vi "Dashboard Main.vi"() -> ()   [LabVIEW 2018]
uses:
  <vilib>/Rock Robotics/WPI/Camera/WPI_CameraExposure Values.ctl
  <vilib>/Rock Robotics/WPI/Camera/WPI_CameraWhite Balance Values.ctl
  <vilib>/Utility/miscctls.llb/LVRowAndColumnTypeDef.ctl
  <vilib>/event_ctls.llb/eventvkey.ctl
  <vilib>/Rock Robotics/Network Tables/NT Read Numeric Array.vi
  <vilib>/Rock Robotics/WPI/Dashboard/WPI_DashboardLogging Global.vi
panel:
  in  "Camera Settings Right":T1={"Frame Rate"=30, "Compression"=30, "Size"=1, "DB Camera Config"=FALSE} {"Frame Rate" scale=1.0..30.0; "Compression" scale=100.0..-1.0; "Size" items=["640x480", "320x240", "160x120"]}
  in  "Camera Name Right":string(combo)="No Camera Selection"
  out "Camera Perf":string
  in  "Camera Settings":T1={"Frame Rate"=30, "Compression"=30, "Size"=1, "DB Camera Config"=FALSE} {"Frame Rate" scale=1.0..30.0; "Compression" scale=100.0..-1.0; "Size" items=["640x480", "320x240", "160x120"]}
  in  "TCP":refnum<k5>
  in  "Rec Mode":enum32{"Stop", "Record", "Playback"}(radio)
  out "Robot IP":string
  out "Image Message":string="Timeout in Camera Communications"
  in  "Dashboard Tab":T2(tab)=enum."Camera"
  in  "Select Auto":string(combo)="Select Autonomous ..."
  out "NT Connection":bool
  out "MotorChart R":cluster{"Numeric":dbl, "Numeric":dbl}(graph)
  out "MotorChart L":cluster{"Numeric":dbl, "Numeric":dbl}(graph)
  out "MotorSliders R":cluster{"MotorSlide1":dbl, "MotorSlide2":dbl} {"MotorSlide2" scale=-1.0..1.0 scale format="%#_2e"; "MotorSlide1" scale=-1.0..1.0 scale format="%#_2e"}
  out "MotorSliders L":cluster{"MotorSlide1":dbl, "MotorSlide2":dbl} {"MotorSlide2" scale=-1.0..1.0 scale format="%#_2e"; "MotorSlide1" scale=-1.0..1.0 scale format="%#_2e"}
  out "Gyro":dbl(knob) scale=0.0..360.0
  out "JS1 Z":dbl(slide) scale=-1.0..1.0 scale format="%#_2e"
  out "JS1 Graph":cluster{"X":dbl, "Y":dbl}[](graph)
  out "JS1 Buttons":T3
  out "JS2 Z":dbl(slide) scale=-1.0..1.0 scale format="%#_2e"
  out "JS2 Graph":cluster{"X":dbl, "Y":dbl}[](graph)
  out "JS2 Buttons":T3
  out "Mode":T4(ring)=enum."Auto Disabled"
  out "Right Camera Perf":cluster{"Bandwidth (Mbps)":dbl, "FPS":dbl}
  out "Camera Image Right":T5(plugin-control)
  in  "DB/String 9":string
  in  "DB/String 8":string
  in  "DB/String 7":string
  in  "DB/String 6":string
  in  "DB/String 5":string
  in  "DB/String 4":string
  in  "DB/String 3":string
  in  "DB/String 2":string
  in  "DB/String 1":string
  in  "DB/String 0":string
  in  "DB/Slider 0":dbl(slide) scale=0.0..5.0
  in  "DB/Slider 1":dbl(slide) scale=0.0..5.0
  in  "DB/Slider 2":dbl(slide) scale=0.0..5.0
  in  "DB/Slider 3":dbl(slide) scale=0.0..5.0
  out "DB/LED 3":bool
  out "DB/LED 2":bool
  out "DB/LED 1":bool
  out "DB/LED 0":bool
  in  "DB/Button 3":bool
  in  "DB/Button 2":bool
  in  "DB/Button 1":bool
  in  "DB/Button 0":bool caption="New Name"
  in  "Camera Settings 3":T8={"Exposure"=enum."Auto", "Exposure (%)"=50.0, "Brightness"=20, "White Balance"=enum."Auto", "Color Temp (K)"=0.0} {"Brightness" min=0 max=100}
  in  "Camera Settings 2":T8={"Exposure"=enum."Auto", "Exposure (%)"=50.0, "Brightness"=20, "White Balance"=enum."Auto", "Color Temp (K)"=0.0} {"Brightness" min=0 max=100}
  in  "Hatch Mover Scale":dbl=0.4 min=0.0 max=1.0 step=0.1
  in  "Elevator Scale":dbl=0.5 min=0.0 max=1.0 step=0.1
  in  "Autonomous Wait":u32=10
  in  "Hatch Extend Setpoint":dbl=0.4 min=0.0 max=1.0 step=0.1 format="%#_1g"
  in  "Hatch Extend Duration":dbl=10.0 min=0.0 max=50.0 step=0.1
  in  "Ball Stop I":dbl=10.0 min=0.0 max=50.0 step=0.1
  in  "Ball Hold Time":dbl=1.0 min=0.0 max=1000.0 step=1.0
  in  "Pivot Left":dbl=0.20000000000000004 min=0.0 max=1.0 step=0.1 format="%#_1g"
  in  "Pivot Right":dbl=0.20000000000000004 min=0.0 max=1.0 step=0.1
  in  "Elevator":dbl=0.7000000000000001 min=0.0 max=1.0 step=0.1 format="%#_3g"
  in  "Elevator Time":dbl=2.0 min=0.0 step=0.1
  in  "Ball":dbl=1.0 min=0.0 max=1.0 step=0.1
  in  "Cheezy Dr Mode":u32=2 max=2 step=1
  in  "MaxSpeedSlow":dbl=0.7
  in  "SlowRate":dbl=1.0
  in  "MaxTurnSlow":dbl=0.65
  in  "MaxTurnRateSlow":dbl=10.0
  in  "SlowModeSettings":i32=2
  in  "Elevator Ball 1":dbl=2.0
  in  "Elevator Ball 2":dbl=2.0
  in  "Elevator Ball 3":dbl=2.0
  in  "Elevator Hatch 1":dbl=2.0
  in  "Elevator Hatch 2":dbl=2.0
  in  "Elevator Hatch 3":dbl=2.0
  in  "Elevator Cargo":dbl=2.0
  in  "Test Slider":dbl(slide) scale=0.0..100.0 scale format="%#_3g"
  in  "On/Off":bool caption="Solenoid"
  in  "Test Name":u16(ring) items=["Select the test to run..."]
  in  "Test Tree":string(tree)
  in  "Motor":cluster{"Value":dbl, "Enable":bool} {"Value" scale=-1.0..1.0 scale format="%#_3g"}
  out "Progress":T9 {"Test Progress" scale=0.0..100.0}
  in  "Rev/Fwd":cluster{"Forward":bool, "Reverse":bool}
  in  "Test Ring":u16(ring) items=["Monochrome", "Color"]
  out "Cmd Status":string
  in  "Execute Command":bool
  in  "Command Params":string[][](table)
  in  "Command Selection":i32(listbox)
  in  "CheckList":i32(listbox)
  out "Tree":string(tree)
  out "Results":T10(array[cluster]) {"Score" format="%#_3g"; "Pixels"."Rectangle"."Numeric 5" format="%#_3g"; "Pixels"."Rectangle"."Numeric 3" format="%#_3g"; "Pixels"."Rectangle"."Numeric 2" format="%#_3g"; "Pixels"."Rectangle"."Numeric" format="%#_3g"; "Normalized"."Rectangle"."Numeric 5" format="%#_2g"; "Normalized"."Rectangle"."Numeric 3" format="%#_2g"; "Normalized"."Rectangle"."Numeric 2" format="%#_2g"; "Normalized"."Rectangle"."Numeric" format="%#_2g"; "Normalized"."Center"."?" format="%#_3g"; "Normalized"."Center"."?" format="%#_3g"; "Distance (ft)" format="%#_3g"}
  out "Camera Image":T5(plugin-control)
  out "Background":bool
  in  "Camera Name":string(combo)="No Camera Selection"
  # "HW"
  # "HW"
  # "Joysticks"
  # "Drive Motors"
  # "Front"
  # "Right"
  # "Left"
  # "Back"
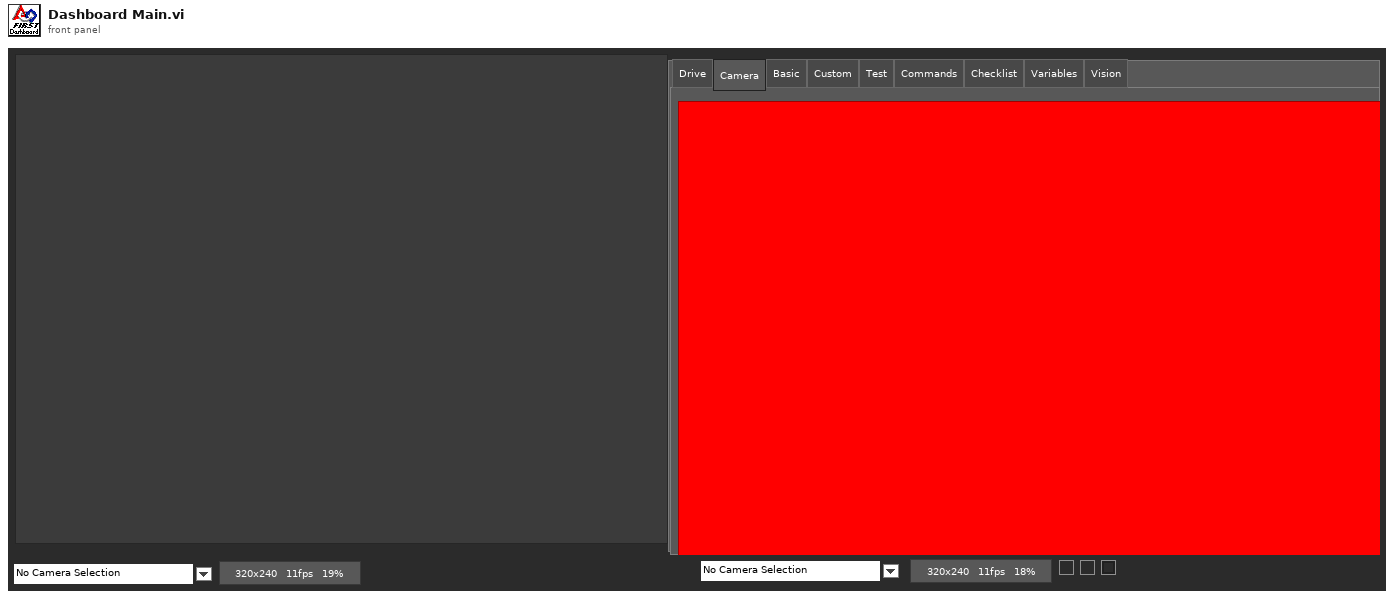
[diagram p1: front panel]
types:
  T1 = cluster{"Frame Rate":i32, "Compression":i32, "Size":u16, "DB Camera Config":bool}
  T2 = enum32{"Drive", "Camera", "Basic", "Custom", "Test", "Commands", "Checklist", "Variables", "Vision"}
  T3 = cluster{bool, bool, bool, bool, bool, bool, bool, bool, bool, bool, bool, bool}
  T4 = enum8{"Tele-Op Disabled", "Tele-Op Enabled", "Auto Disabled", "Auto Enabled", "Test Disabled", "Test Enabled", "Disconnected", "No Code", "E-Stop"}
  T5 = typedef "IMAQ Image.ctl" = refnum<image>
  T6 = typedef "WPI_CameraExposure Values.ctl" = enum16{"Auto", "Flicker-free 50 Hz", "Flicker-free 60 Hz", "Hold current", "Custom"}
  T7 = typedef "WPI_CameraWhite Balance Values.ctl" = enum16{"Auto", "Fixed indoor", "Fixed outdoor 1", "Fixed outdoor 2", "Fixed fluorescent 1", "Fixed fluorescent 2", "Hold current", "Custom"}
  T8 = cluster{"Exposure":T6, "Exposure (%)":dbl, "Brightness":i32, "White Balance":T7, "Color Temp (K)":dbl}
  T9 = cluster{"Test Progress":u8, "Test Progress Text":string}
  T10 = cluster{"Distance (ft)":dbl, "Score":dbl, "Normalized":cluster{"Center":cluster{dbl, dbl}, "Rectangle":cluster{"Numeric":dbl, "Numeric 2":dbl, "Numeric 3":dbl, "Numeric 5":dbl}}, "Pixels":cluster{"Center":cluster{dbl, dbl}, "Rectangle":cluster{"Numeric":dbl, "Numeric 2":dbl, "Numeric 3":dbl, "Numeric 5":dbl}}}[]
  T11 = typedef "Image Type" = u32
  T12 = cluster{"Save Path":path, "Interval (s)":dbl, "Keep":i32}
  T13 = enum32{"Drive", "Camera", "Basic", "Custom", "Test", "Commands", "Checklist", "Variables"}
  T14 = cluster{"IDs":cluster{"RPC field ID":u16, "Unique ID":u16}, "String":string}
  T15 = cluster{"Error Strings":string, "Disable Counts":cluster{u16, u16}, "Rail Faults":cluster{u16, u16, u16}, "Robot IP":string, "DB Mode":u8, "Event Info":cluster{"Name":string, "Type":u8, "Number":u16, "Replay":u8}}
  T16 = cluster{"Storage":cluster{"Disk Free":u64, "RAM Block":u32, "RAM free":u32}, "CPU Utilization":cluster{"CPU % ISR":sgl, "CPU % Time Crit":sgl, "CPU % Timed Str":sgl, "CPU % High":sgl, "CPU % Above":sgl, "CPU % Normal":sgl, "CPU % Low":sgl}, "CAN":cluster{"% Bus Utilization":sgl, "Bus Off Cnt":u32, "TX_FIFO Full Cnt":u32, "Receive Error Cnt":u8, "Transmit Error Cnt":u8}, "HID":cluster{"HID Outputs":u32, "Rumble Low":u16, "Rumble High":u16}[]}
  T17 = cluster{"Status bits":cluster{"Test Mode":bool, "Autonomous":bool, "Enabled":bool, "Code Start":bool, "Brownout":bool, "Reserved 2":bool, "Reserved 3":bool, "E-Stop":bool}, "Code Trace":cluster{"Disabled":bool, "TeleOp":bool, "Auto":bool, "Test":bool}, "Controller Type":enum16{"unknown", "cRIO", "roboRio"}, "Code?":enum16{"unknown", "noCode", "code"}, "Battery V":dbl}
  T18 = cluster{"Control Bits":cluster{"TestMode":bool, "Autonomous":bool, "Enabled":bool, "FMS Present":bool, bool, bool, bool, "E-Stop":bool}, "Team Station ":u8, "Countdown":sgl, "Joystick Values":cluster{"Axes":dbl[], "Buttons":bool[], "POVs":i16[]}[]}
  T19 = cluster{"Axes":dbl[], "Buttons":bool[], "POVs":i16[]}[]
  T20 = cluster{"Axes":dbl[], "Buttons":bool[], "POVs":i16[]}
  T21 = cluster{"Buttons[0]":bool, "Buttons[1]":bool, "Buttons[2]":bool, "Buttons[3]":bool, "Buttons[4]":bool, "Buttons[5]":bool, "Buttons[6]":bool, "Buttons[7]":bool, "Buttons[8]":bool, "Buttons[9]":bool, "Buttons[10]":bool, "Buttons[11]":bool}
  T22 = cluster{"Camera Image":refnum<vi>, "Dashboard Tab":refnum<vi>, "Background":refnum<vi>, "Rec Mode":refnum<vi>, "Test Slider":refnum<vi>, "On/Off ":refnum<vi>, "Test Ring":refnum<vi>, "Rev/Fwd":refnum<vi>, "Test Name":refnum<vi>, "Motor":refnum<vi>, "Progress":refnum<vi>, "CheckList":refnum<vi>, "Tree":refnum<vi>, "Test Tree":refnum<vi>, "Command Params":refnum<vi>, "Command Selection":refnum<vi>, "Execute Command":refnum<vi>, "Cmd Status":refnum<vi>, "Camera Settings":refnum<vi>, "Camera Name":refnum<vi>, "Camera Perf":refnum<vi>, "Camera Settings Right":refnum<vi>, "Camera Name Right":refnum<vi>, "Camera Image Right":refnum<vi>}
  T23 = cluster{"Global Rectangle":i32[], "Contours":cluster{"Contour Type":u32, "ROI Type":u32, "Points":i32[]}[]}
  T24 = cluster{"Camera Name":string, string, "Saved DB Images Info":cluster{"Save Path":path, "Interval (s)":dbl, "Keep":i32}}
  T25 = cluster{"Camera Name Right":string, string, "Saved DB Images Info":cluster{"Save Path":path, "Interval (s)":dbl, "Keep":i32}}
  T26 = cluster{"Operation":enum16{"Update", "Clear"}, "Color Box":u32}[]
  T27 = typedef "eventvkey.ctl" = enum16{"ASCII", "Enter", "Return", "Shift", "Ctrl", "Alt", "Cmd", "Opt", "Caps", "NumLock", "Clear", "Break", "Up", "Down", "Left", "Right", "Insert", "Delete", "Home", "End", "PageUp", "PageDown", "Escape", "Help", "Pause", "ScrollLock", "F1", "F2", "F3", "F4", "F5", "F6", "F7", "F8", "F9", "F10", "F11", "F12", "F13", "F14", "F15", "F16", "F17", "F18", "F19", "F20", "F21", "F22", "F23", "F24", "Play", "VolumeUp", "VolumeDown", "Mute", "Two Byte Char"}
  T28 = cluster{"Image Size":bool, "Image Type":bool, "Pixel Value":bool, "ROI Information":bool, "Zoom Factor":bool}
  T29 = cluster{"Operation":enum16{"Update", "Clear"}, "Color Box":u32}
  T30 = typedef "LVRowAndColumnTypeDef.ctl" = cluster{"Row":i32, "Column":i32}
  T31 = cluster{"Shift":bool, "Ctrl":bool, "Alt":bool, "Cmd":bool, "Opt":bool}
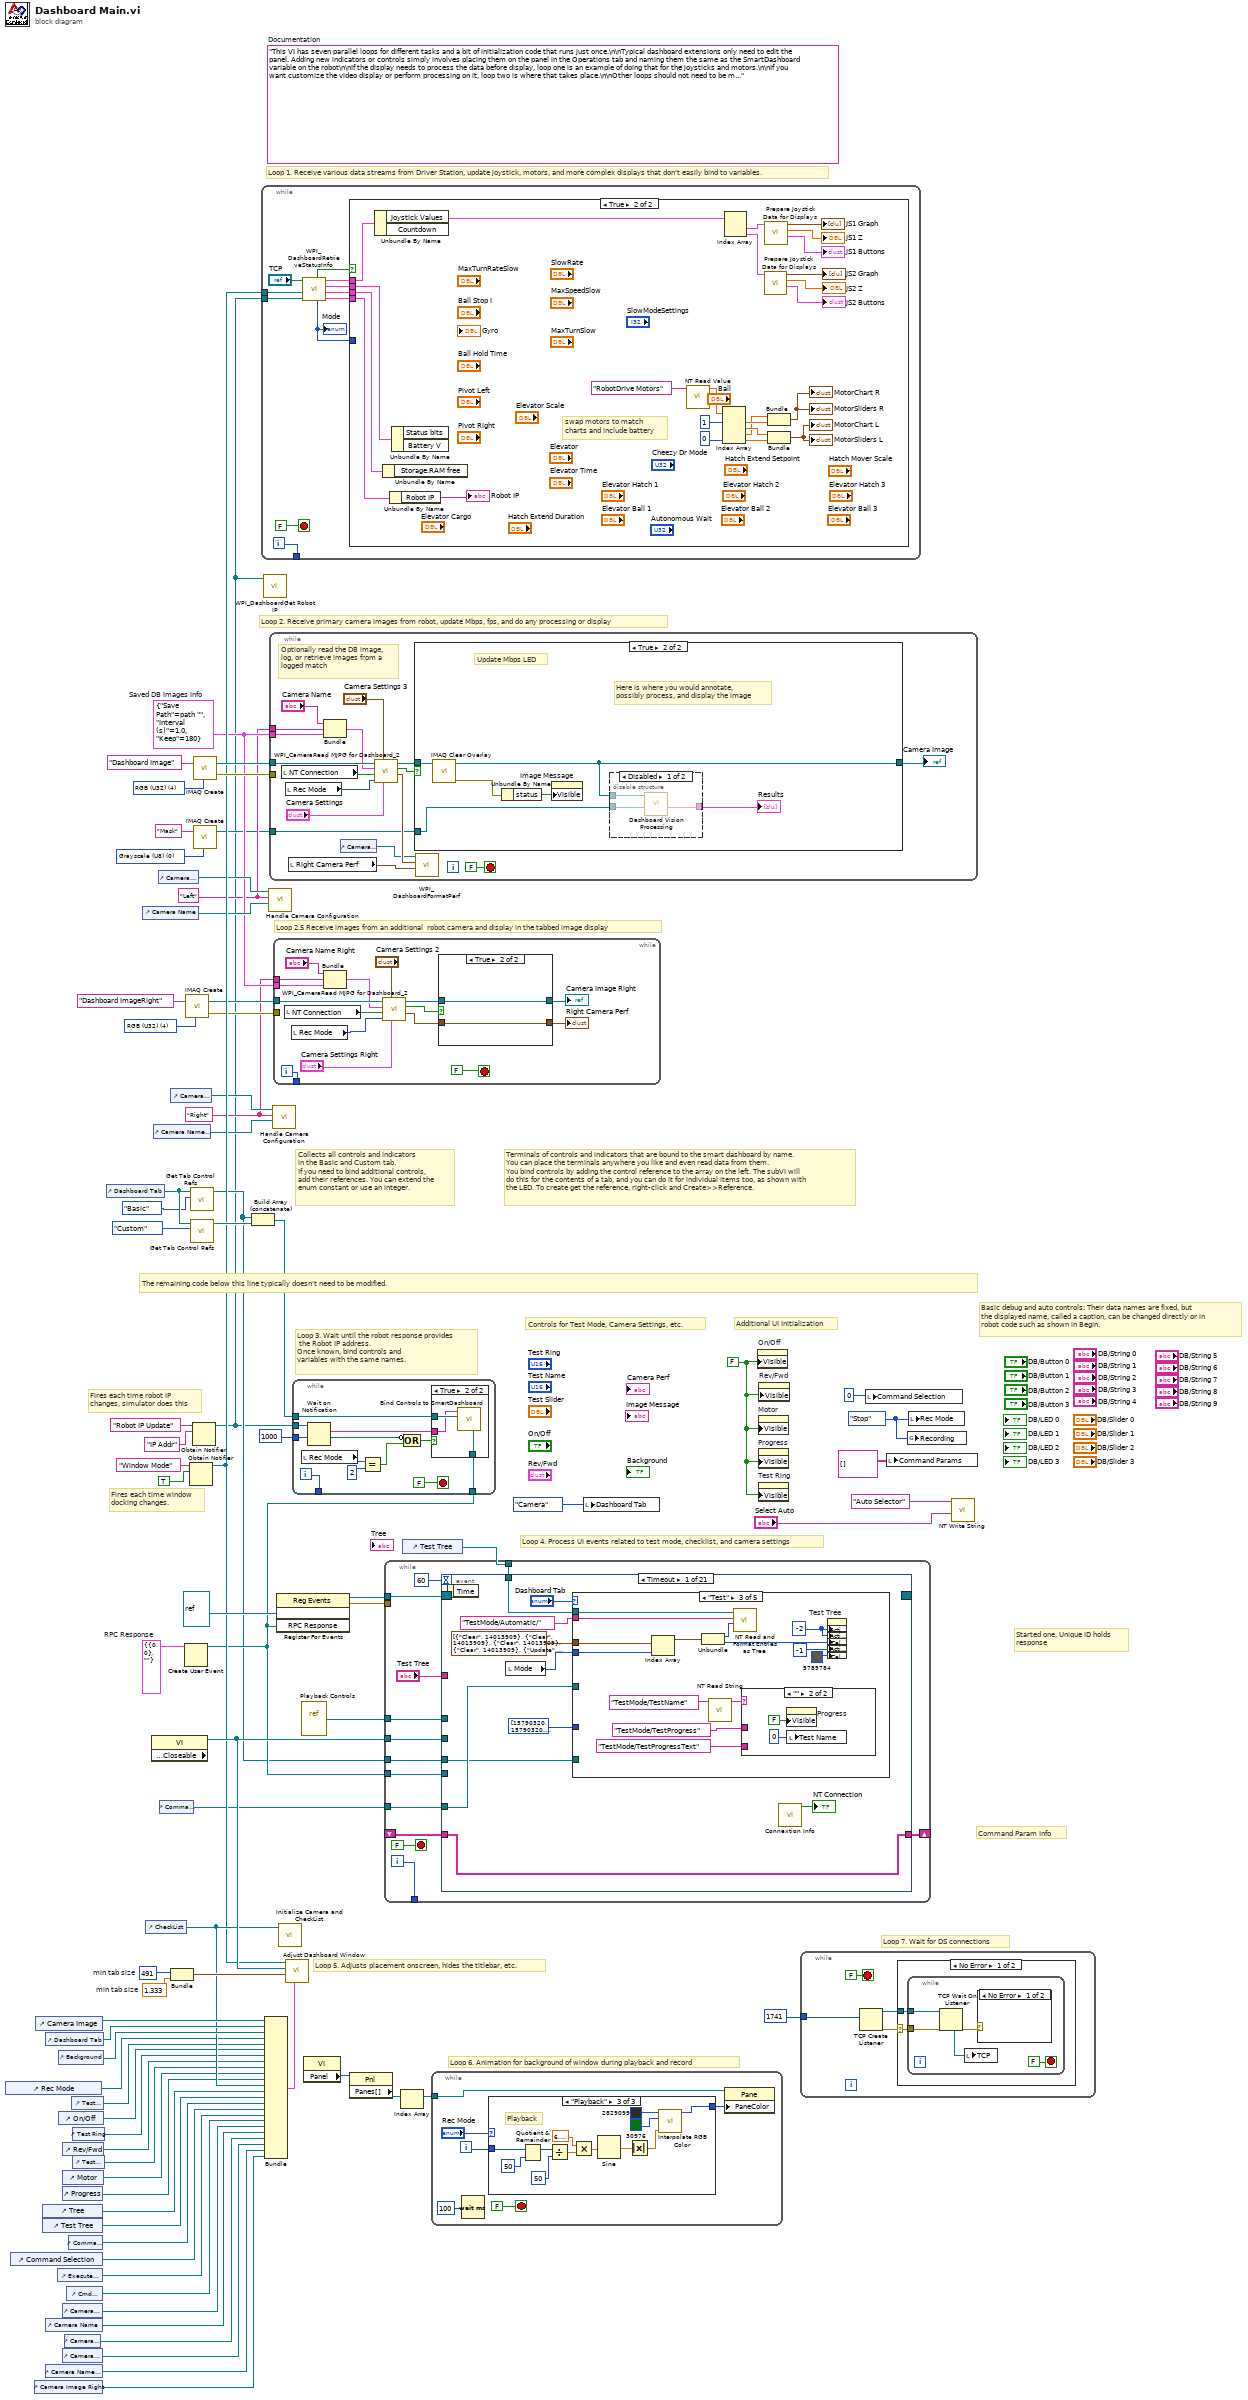
[diagram p0: block diagram]
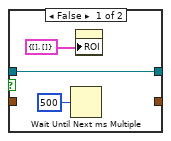
[diagram p2: hidden frame]
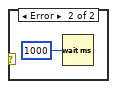
[diagram p3: hidden frame]
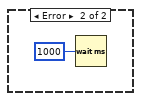
[diagram p4: hidden frame]
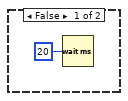
[diagram p5: hidden frame]
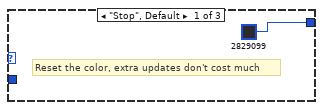
[diagram p6: hidden frame]
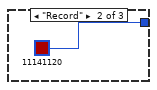
[diagram p7: hidden frame]
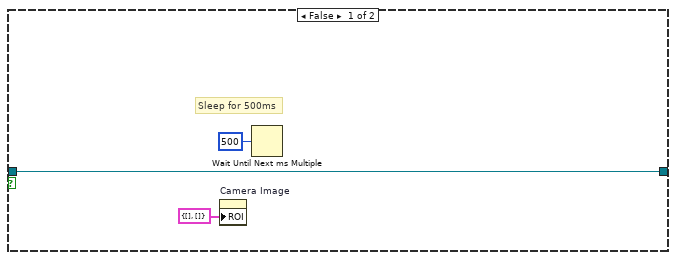
[diagram p9: hidden frame]
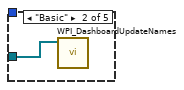
[diagram p12: hidden frame]
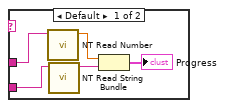
[diagram p13: hidden frame]
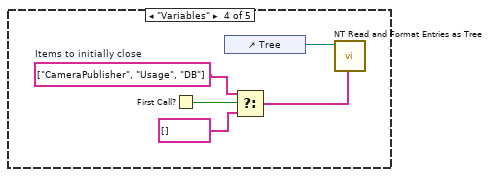
[diagram p14: hidden frame]
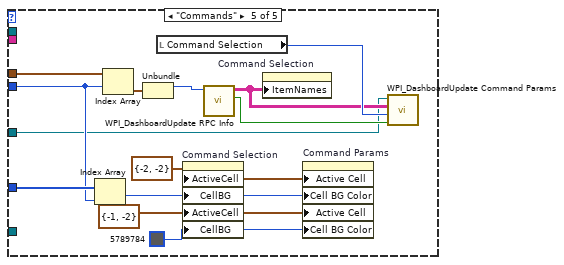
[diagram p15: hidden frame]
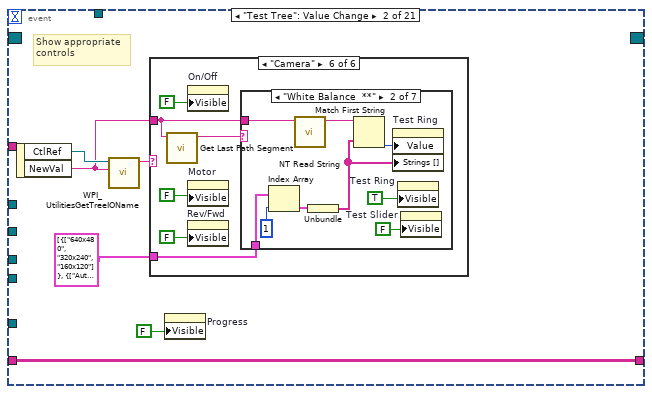
[diagram p16: hidden frame]
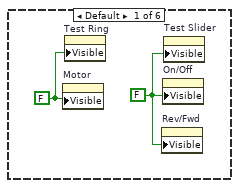
[diagram p17: hidden frame]
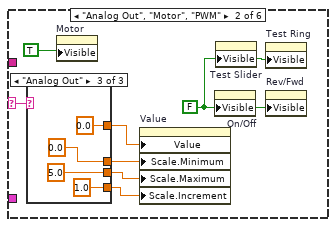
[diagram p18: hidden frame]
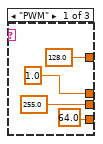
[diagram p19: hidden frame]
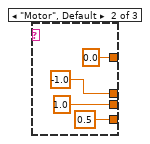
[diagram p20: hidden frame]
diagram:
  w3 = T11 0 items=["Grayscale (U8)", "Grayscale (I16)", "Grayscale (SGL)", "Complex (CSG)", "RGB (U32)", "HSL (U32)", "RGB (U64)"] ("Image Type")
  w7 = T12 {"Save Path"=path "", "Interval (s)"=1.0, "Keep"=180}  # Saved DB Images Info
  w6 = "Right"
  w5 = "Left"
  w17 = T11 4 items=["Grayscale (U8)", "Grayscale (I16)", "Grayscale (SGL)", "Complex (CSG)", "RGB (U32)", "HSL (U32)", "RGB (U64)"] ("Image Type")
  w33 = T14 {"IDs"={"RPC field ID"=0, "Unique ID"=0}, "String"=""}  # RPC Response
  w55 = 491  # min tab size
  w54 = 1.333  # min tab size
  w62 = enum32{"Stop", "Record", "Playback"}."Stop" ("Rec Mode")
  w39 = FALSE ("Visible")
  (unwired) "This VI has seven parallel loops for different tasks and a bit of initialization code that runs just once.\n\nTypical dashboard extensions only need to edit the panel. Adding new indicators or controls simply involves placing them on the panel in the Operations tab and naming them the same as the SmartDashboard variable on the robot\n\nIf the display needs to process the data before display, loop one is an example of doing that for the joysticks and motors.\n\nIf you want customize the video display or perform processing on it, loop two is where that takes place.\n\nOther loops should not need to be modified. They are pretty standard, and document the task they perform."  # Documentation
  w79 = T11 4 items=["Grayscale (U8)", "Grayscale (I16)", "Grayscale (SGL)", "Complex (CSG)", "RGB (U32)", "HSL (U32)", "RGB (U64)"] ("Image Type")
  # "Loop 2.5 Receive images from an additional  robot camera and display in the tabbed image display"
  # "Command Param Info"
  # "Started one, Unique ID holds\nresponse"
  # "Loop 7. Wait for DS connections"
  # "Basic debug and auto controls: Their data names are fixed, but\nthe displayed name, called a caption, can be changed directly or in\nrobot code such as shown in Begin."
  # "Controls for Test Mode, Camera Settings, etc."
  # "Additional UI Initialization"
  # "Loop 6. Animation for background of window during playback and record"
  # "Fires each time robot IP\nchanges, simulator does this"
  # "Fires each time window\ndocking changes."
  # "Collects all controls and indicators\nin the Basic and Custom tab.\nIf you need to bind additional controls,\nadd their references. You can extend the\nenum constant or use an integer."
  # "The remaining code below this line typically doesn't need to be modified."
  # "Loop 4. Process UI events related to test mode, checklist, and camera settings"
  # "Terminals of controls and indicators that are bound to the smart dashboard by name.\nYou can place the terminals anywhere you like and even read data from them.\nYou bind controls by adding the control reference to the array on the left. The subVI will\ndo this for the contents of a tab, and you can do it for individual items too, as shown with\nthe LED. To create get the reference, right-click and Create>>Reference."
  # "Loop 3. Wait until the robot response provides\n the Robot IP address.\nOnce known, bind controls and\nvariables with the same names."
  # "Loop 5. Adjusts placement onscreen, hides the titlebar, etc."
  # "Loop 1. Receive various data streams from Driver Station, update joystick, motors, and more complex displays that don't easily bind to variables."
  # "Loop 2. Receive primary camera images from robot, update Mbps, fps, and do any processing or display"
  n1 = control-ref of="Rec Mode"() -> (w45:refnum<vi>)
  n2 = control-ref of="Command Selection"() -> (w32:refnum<vi>)
  n3 = control-ref of="Camera Image Right"() -> (w10:refnum<vi>)
  n4 = control-ref of="Camera Image"() -> (w57:refnum<vi>)
  n5 = control-ref of="Tree"() -> (w49:refnum<vi>)
  n6 = control-ref of="Test Tree"() -> (w48:refnum<vi>)
  n7 = control-ref of="Dashboard Tab"() -> (w56:refnum<vi>)
  n8 = control-ref of="Camera Name"() -> (w23:refnum<vi>)
  n9 = control-ref of="Camera Name Right"() -> (w11:refnum<vi>)
  n10 = control-ref of="Execute Command"() -> (w34:refnum<vi>)
  n11 = control-ref of="Background"() -> (w52:refnum<vi>)
  n12 = control-ref of="On/Off"() -> (w43:refnum<vi>)
  n13 = control-ref of="Progress"() -> (w40:refnum<vi>)
  n14 = control-ref of="Camera Settings"() -> (w24:refnum<vi>)
  n15 = control-ref of="Camera Settings Right"() -> (w12:refnum<vi>)
  n16 = control-ref of="Rev/Fwd"() -> (w41:refnum<vi>)
  n17 = control-ref of="Motor"() -> (w46:refnum<vi>)
  n18 = control-ref of="Camera Perf"() -> (w22:refnum<vi>)
  n19 = control-ref of="Cmd Status"() -> (w28:refnum<vi>)
  n20 = control-ref of="Command Params"() -> (w35:refnum<vi>)
  n21 = control-ref of="Test Slider"() -> (w44:refnum<vi>)
  n22 = control-ref of="Test Ring"() -> (w42:refnum<vi>)
  n23 = control-ref of="Test Name"() -> (w47:refnum<vi>)
  n24 = control-ref of="Dashboard Tab"() -> (w60:refnum<vi>)
  n25 = control-ref of="Camera Name"() -> (w25:refnum<vi>)
  n26 = control-ref of="CheckList"() -> (w50:refnum<vi>)
  n27 = property class="VI" props=["Front Panel.Closeable"]() -> (reference out=w61:refnum<vi>)  [unwired: 2 in, 2 out]
  n28 = control-ref of="Camera Name Right"() -> (w13:refnum<vi>)
  n29 = control-ref of="Camera Settings"() -> (w26:refnum<vi>)
  n30 = control-ref of="Command Params"() -> (w27:refnum<vi>)
  n31 = control-ref of="Camera Settings Right"() -> (w14:refnum<vi>)
  n32 = Bundle("min tab size"=w55, "min tab size"=w54) -> (w53:cluster{"min tab size":i32, "min tab size":dbl})  [unwired: 1 in]
  n33 = Create User Event(user event datatype=w33) -> (user event=w29:refnum<user-event>)  [unwired: 1 in, 1 out]
  n34 = call "IMAQ Create"("Image Name"="Dashboard ImageRight", "Image Type"=w17) -> ("New Image"=w16:T5, "error out"=w15:errorcluster)  [unwired: 2 in, 1 out]
  n35 = Obtain Notifier(name (unnamed)="Window Mode", notification data type=TRUE) -> (notifier out=w38:refnum<notifier>)  [unwired: 2 in, 2 out]
  n36 = call <vilib>:"Get Tab Control Refs.vi"("Page Index"=T13."Basic" ("Dashboard Tab"), "TabControl in"=w60) -> ("ControlsOnPage"=w21:refnum<vi>[])  [unwired: 9 in]
  n37 = call <vilib>:"Get Tab Control Refs.vi"("Page Index"=T13."Custom" ("Dashboard Tab"), "TabControl in"=w60) -> ("ControlsOnPage"=w59:refnum<vi>[])  [unwired: 9 in]
  n38 = Obtain Notifier(name (unnamed)="Robot IP Update", notification data type="IP Addr" ("name (unnamed)")) -> (notifier out=w1:refnum<notifier>)  [unwired: 2 in, 2 out]
  n39 = call "IMAQ Create"("Image Name"="Dashboard Image", "Image Type"=w79) -> ("New Image"=w77:T5, "error out"=w76:errorcluster)  [unwired: 2 in, 1 out]
  n40 = call "IMAQ Create"("Image Name"="Mask", "Image Type"=w3) -> ("New Image"=w2:T5)  [unwired: 2 in, 2 out]
  n41 = Build Array (concatenate)(w21, w59) -> (w58:refnum<vi>[])
  n42 = while {
    tunnel: [w89] -> _
    tunnel: w1 -> [w83]
    tunnel: w38 -> [w80]
    i -> [w89]
    stop <- FALSE stop-if-true
    n43 = call <vilib>:"WPI_DashboardRetrieveStatusInfo.vi"("Binding Refnum"=w83, "Window Mode Notifier"=w80, "TCP Cnx"="TCP") -> ("Power and Errors"=w84:T15, "Robot Metrics"=w87:T16, "Status Info"=w88:T17, "Control Info"=w85:T18, "Robot Mode"=w82:T4, "Process?"=w86:bool)  [unwired: 3 in]
    "Mode" <- w82
    n44 = case shown="True" w86 {
      tunnel: w88 -> [_ w115]
      tunnel: w87 -> [_ w114]
      tunnel: w85 -> [_ w113]
      tunnel: w84 -> [_ w112]
      tunnel: w82 -> [_ _]
      frame False {
        n45 = Wait (ms)(milliseconds to wait=u32 20) -> ()  [unwired: 1 out]
      }
      frame True {
        # "swap motors to match\ncharts and include battery"
        n46 = Unbundle By Name(w113) -> ("Joystick Values"=w103:T19)  [unwired: 1 out]
        n47 = Unbundle By Name(w114) -> ()  [unwired: 1 out]
        n48 = Unbundle By Name(w112) -> ("Robot IP"=→"Robot IP":string)
        n49 = Unbundle By Name(w115) -> ()  [unwired: 2 out]
        n50 = call-poly <vilib>:"NT Read Value.vi"("Name"="RobotDrive Motors") -> ("Numeric Array"=w93:dbl[])  [unwired: 9 in, 1 out]
        n51 = Index Array(array=w93, index #1=1, index #4=0) -> (element #1=w107:dbl, element #2=w108:dbl, element #3=w106:dbl, element #4=w111:dbl)  [unwired: 2 in]
        n52 = Index Array(array=w103) -> (element #1=w102:T20, element #2=w98:T20)  [unwired: 2 in]
        n53 = call "Prepare Joystick Data for Displays.vi"("Joystick Values"=w98) -> ("Buttons"=→"JS2 Buttons":T21, "Z Axis"=→"JS2 Z":dbl, "Cartesian Data"=→"JS2 Graph":cluster{"X axis":dbl, "X axis":dbl}[])  [unwired: 8 in]
        n54 = call "Prepare Joystick Data for Displays.vi"("Joystick Values"=w102) -> ("Buttons"=→"JS1 Buttons":T21, "Z Axis"=→"JS1 Z":dbl, "Cartesian Data"=→"JS1 Graph":cluster{"X axis":dbl, "X axis":dbl}[])  [unwired: 8 in]
        n55 = Bundle("Numeric"=w106, "Numeric"=w107) -> (→"MotorChart R" →"MotorSliders R":cluster{"Numeric":dbl, "Numeric":dbl})  [unwired: 1 in]
        n56 = Bundle("Numeric"=w108, "Numeric"=w111) -> (→"MotorChart L" →"MotorSliders L":cluster{"Numeric":dbl, "Numeric":dbl})  [unwired: 1 in]
      }
    }
  }
  n57 = call <vilib>:"WPI_DashboardGet Robot IP.vi"("Notifier in"=w1) -> ()  [unwired: 11 in]
  n58 = Bundle("Camera Image"=w57, "Dashboard Tab"=w56, "Background"=w52, "Rec Mode"=w45, "Test Slider"=w44, "On/Off"=w43, "Test Ring"=w42, "Rev/Fwd"=w41, "Test Name"=w47, "Motor"=w46, "Progress"=w40, "CheckList"=w50, "Tree"=w49, "Test Tree"=w48, "Command Params"=w35, "Command Selection"=w32, "Execute Command"=w34, "Cmd Status"=w28, "Camera Settings"=w24, "Camera Name"=w23, "Camera Perf"=w22, "Camera Settings Right"=w12, "Camera Name Right"=w11, "Camera Image Right"=w10) -> (w51:T22)  [unwired: 1 in]
  n59 = call "Handle Camera Configuration.vi"("CameraNameRef"=w25, "Display Name"=w5, "ClusterRef"=w26) -> ()  [unwired: 9 in]
  n60 = while {
    tunnel: w77 -> [w131]
    tunnel: w76 -> [_]
    tunnel: w7 -> [w124]
    tunnel: w5 -> [w121]
    tunnel: w2 -> [w117]
    stop <- FALSE stop-if-true
    # "Optionally read the DB image,\nlog, or retrieve images from a\nlogged match"
    n61 = local read "NT Connection"() -> (w125:bool)
    n62 = local read "Rec Mode"() -> (w128:enum32{"Stop", "Record", "Playback"})
    n63 = local read "Right Camera Perf"() -> (w119:cluster{"Bandwidth (Mbps)":dbl, "FPS":dbl})
    n64 = Bundle("Camera Name"="Camera Name", w121, "Saved DB Images Info"=w124) -> (w123:T24)  [unwired: 1 in]
    n65 = control-ref of="Camera Perf"() -> (w118:refnum<vi>)
    n66 = call <vilib>:"WPI_CameraRead MJPG for Dashboard_2.vi"("Camera Settings"="Camera Settings", "Camera Settings 2"="Camera Settings 3", "Rec Mode"=w128, "NT Connection"=w125, "Capture Info"=w123, "Image in"=w131) -> ("perf info"=w120:cluster{"Bandwidth (Mbps)":dbl, "fps":dbl}, "Active"=w129:bool, "Image\\ out"=w130:T5)  [unwired: 3 in]
    n67 = case shown="True" w129 {
      tunnel: w130 -> [w134 w139]
      tunnel: [w134 w138] -> w126
      tunnel: w117 -> [_ w137]
      frame False {
        # "Sleep for 500ms"
        n68 = property on="Camera Image" class="ImageControl"("ROI"=T23 {"Global Rectangle"=[], "Contours"=[]}) -> ()  [unwired: 2 in, 2 out]
        n69 = Wait Until Next ms Multiple(millisecond multiple=u32 500) -> ()  [unwired: 1 out]
      }
      frame True {
        # "Here is where you would annotate,\npossibly process, and display the image"
        # "Update Mbps LED"
        n70 = call "IMAQ Clear Overlay"("Image"=w139) -> ("error out"=w140:errorcluster, "Image Out"=w138:T5)  [unwired: 2 in, 7 out]
        n71 = Unbundle By Name(w140) -> ("status"=w141:bool)
        n72 = property on="Image Message" class="Str"("Visible"=w141) -> ()  [unwired: 2 in, 2 out]
        n73 = disable-structure shown="Disabled" {
          disable-tunnel: w138 -> [w144 _]
          disable-tunnel: w137 -> [w143 _]
          disable-tunnel: [w142 _] -> w136
          frame Disabled {
            n74 = call "Dashboard Vision Processing.vi"("Image 2"=w143, "Image"=w144) -> ("Results"=w142:T10)  [unwired: 8 in, 1 out]
          }
          frame Enabled {
          }
        }
        "Results" <- w136
      }
    }
    "Camera Image" <- w126
    n75 = call <vilib>:"WPI_DashboardFormatPerf.vi"("Right Camera Perf"=w119, "Performance"=w120, "String in"=w118) -> ()  [unwired: 9 in]
  }
  n76 = call "Handle Camera Configuration.vi"("CameraNameRef"=w13, "Display Name"=w6, "ClusterRef"=w14) -> ()  [unwired: 9 in]
  n77 = while {
    tunnel: w16 -> [w160]
    tunnel: w15 -> [_]
    tunnel: [w155] -> _
    tunnel: w7 -> [w151]
    tunnel: w6 -> [w148]
    i -> [w155]
    stop <- FALSE stop-if-true
    n78 = local read "NT Connection"() -> (w152:bool)
    n79 = local read "Rec Mode"() -> (w159:enum32{"Stop", "Record", "Playback"})
    n80 = Bundle("Camera Name Right"="Camera Name Right", w148, "Saved DB Images Info"=w151) -> (w150:T25)  [unwired: 1 in]
    n81 = call <vilib>:"WPI_CameraRead MJPG for Dashboard_2.vi"("Camera Settings"="Camera Settings Right", "Camera Settings 2"="Camera Settings 2", "Rec Mode"=w159, "NT Connection"=w152, "Capture Info"=w150, "Image in"=w160) -> ("perf info"=w146:cluster{"Bandwidth (Mbps)":dbl, "fps":dbl}, "Active"=w154:bool, "Image\\ out"=w157:T5)  [unwired: 3 in]
    n82 = case shown="True" w154 {
      tunnel: w157 -> [w162 w165]
      tunnel: [w162 w165] -> w153
      tunnel: [_ w164] -> w147
      tunnel: w146 -> [_ w164]
      frame False {
        n83 = Wait Until Next ms Multiple(millisecond multiple=u32 500) -> ()  [unwired: 1 out]
        n84 = property on="Camera Image Right" class="ImageControl"("ROI"=T23 {"Global Rectangle"=[], "Contours"=[]}) -> ()  [unwired: 2 in, 2 out]
      }
      frame True {
      }
    }
    "Camera Image Right" <- w153
    "Right Camera Perf" <- w147
  }
  n85 = register-events(refnum<vi> refnum, w29) -> (reference out=w66:refnum<event-registration>, error out=w65:errorcluster)  [unwired: 2 in]
  n86 = call "Initialize Camera and CheckList.vi"("ListBox in"=w50) -> ()  [unwired: 11 in]
  n87 = call "Adjust Dashboard Window.vi"("Sizing Refnums"=w51, "Size Constraints"=w53, "VI"=w61, "WIn Mode"=w38) -> ()  [unwired: 8 in]
  n88 = while {
    tunnel: w58 -> [w177]
    tunnel: w1 -> [w175]
    tunnel: [w173] -> _
    tunnel: u32 1000 ("milliseconds to wait") -> [w172]
    tunnel: w29 -> [w166]
    i -> [w173]
    stop <- FALSE stop-if-true
    n89 = local read "Rec Mode"() -> (w168:enum32{"Stop", "Record", "Playback"})
    n90 = Wait on Notification(notifier=w175, timeout in ms (-1)=w172) -> (notification=w174:string, timed out?=w170:bool)  [unwired: 2 in, 2 out]
    n91 = Equal?(x=w168, y=u16 2 ("Rec Mode")) -> (x = y?=w169:bool)
    n92 = Compound Arithmetic op=OR(invert w170, w169) -> (w171:bool)
    n93 = case shown="True" w171 {
      tunnel: w177 -> [_ w180]
      tunnel: w174 -> [_ w179]
      tunnel: w166 -> [_ w178]
      frame False {
      }
      frame True {
        n94 = call <vilib>:"Bind Controls to SmartDashboard.vi"("RPC ref"=w178, "Bound Control Refs"=w180, "Server IP Address"=w179) -> ()  [unwired: 9 in]
      }
    }
  }
  n95 = vi-ref "Playback Controls.vi"() -> (w67:refnum<vi>)
  n96 = property class="VI"() -> ("Panel"=w69:refnum<vi>)  [unwired: 2 in, 2 out]
  n97 = property class="Pnl"(reference=w69) -> ("Panes[]"=w70:refnum<vi>[])  [unwired: 1 in, 2 out]
  n98 = Index Array(array=w70) -> (element=w68:refnum<vi>)  [unwired: 1 in]
  n99 = control-ref of="Test Tree"() -> (w71:refnum<vi>)
  n100 = while {
    tunnel: [w190] -> _
    tunnel: w71 -> [w189]
    tunnel: w67 -> [w188]
    tunnel: w66 -> [w187]
    tunnel: w65 -> [_]
    tunnel: w61 -> [w186]
    tunnel: w29 -> [w185]
    tunnel: w27 -> [w184]
    shift-right: [w183] -> _
    shift-left: _ -> [w182]
    tunnel: w21 -> [w181]
    i -> [w190]
    stop <- FALSE stop-if-true
    n101 = event shown="[0] Timeout" {
      selector: w187 -> [_ _ _ _ _ _ _ _ _ _ _ _ _ _ _ _ _ _ _ _ _]
      dyn-events: [_ _ _ _ _ _ _ _ _ _ _ _ _ _ _ _ w450 _ _ _ _] -> _
      timeout: u32 60 ("milliseconds to wait") -> [_ _ _ _ _ _ _ _ _ _ _ _ _ _ _ _ _ _ _ _ _]
      tunnel: w189 -> [w202 _ _ _ _ _ _ _ _ _ _ _ _ _ _ _ _ _ _ _ _]
      tunnel: "Test Tree" -> [_ _ _ _ _ _ _ _ _ _ _ w417 w425 w427 w431 w439 _ _ _ _ _]
      tunnel: w188 -> [_ _ _ _ _ _ _ _ _ _ _ _ _ _ _ _ w452 _ w470 _ _]
      tunnel: w186 -> [_ _ _ _ _ _ _ _ _ _ _ _ _ _ _ _ w448 _ _ _ _]
      tunnel: w185 -> [_ _ _ _ _ _ _ _ _ _ _ _ _ _ _ _ w446 _ _ _ _]
      tunnel: w184 -> [w197 _ _ _ _ _ w368 _ _ _ _ _ _ _ _ _ _ _ _ _ _]
      tunnel: [w196 w245 w347 w352 w361 w365 w366 w375 w385 w392 w404 w416 w423 w426 w430 w438 w445 w465 w467 w471 w484] -> w183
      tunnel: w182 -> [w196 w245 w347 w352 w361 w365 w366 _ _ w392 w404 w416 w423 w426 w430 w438 w445 w465 w467 w471 w484]
      tunnel: w181 -> [w194 _ _ _ _ _ _ _ _ _ _ _ _ _ _ _ _ _ _ _ _]
      event Timeout {
        n102 = event-data() -> ()  [unwired: 1 in, 1 out]
        n103 = local read "Mode"() -> (w199:T4)
        n104 = case shown="\"Test\"" "Dashboard Tab" {
          tunnel: w202 -> [_ _ w218 _ _]
          tunnel: "TestMode/Automatic/" ("Name Pattern") -> [_ _ w217 _ _]
          tunnel: T26 [{"Operation"=enum."Clear", "Color Box"=14013909}, {"Operation"=enum."Clear", "Color Box"=14013909}, {"Operation"=enum."Clear", "Color Box"=14013909}, {"Operation"=enum."Clear", "Color Box"=14013909}, {"Operation"=enum."Update", "Color Box"=14013909}, {"Operation"=enum."Update", "Color Box"=16777215}, {"Operation"=enum."Clear", "Color Box"=14013909}, {"Operation"=enum."Clear", "Color Box"=14013909}, {"Operation"=enum."Clear", "Color Box"=14013909}] -> [_ _ w210 _ w238]
          tunnel: w199 -> [_ _ w209 _ w237]
          tunnel: u32[] [15790320, 15790320, 15790320, 15790320, 16777215, 16777215, 15790320, 15790320, 15790320] -> [_ _ _ _ w243]
          tunnel: w197 -> [_ _ _ _ w231]
          tunnel: w194 -> [_ w204 _ _ _]
          frame "Custom", Default {
          }
          frame "Basic" {
            n105 = call <vilib>:"WPI_DashboardUpdateNames.vi"("Controls on Tab"=w204) -> ()  [unwired: 11 in]
          }
          frame "Test" {
            w216 = -2 ("Active Item:Row Number")
            n106 = Index Array(array=w210, index=w209) -> (element=w211:T29)
            n107 = Unbundle(w211) -> ("Operation"=w212:enum16{"Update", "Clear"}, "Color Box"=w213:u32)
            n108 = call <vilib>:"NT Read String.vi"("Name"="TestMode/TestName") -> ("String"=w207:string)  [unwired: 9 in, 1 out]
            n109 = call <vilib>:"NT Read and Format Entries as Tree.vi"("Operation"=w212, "Name Pattern"=w217, "Tree Refnum"=w218) -> ()  [unwired: 7 in, 2 out]
            n110 = case shown="\"\"" w207 {
              tunnel: "TestMode/TestProgress" ("Name") -> [w220 _]
              tunnel: "TestMode/TestProgressText" ("Name") -> [w219 _]
              frame Default {
                n111 = call <vilib>:"NT Read Number.vi"("Name"=w220) -> ("Numeric"=w221:dbl)  [unwired: 9 in, 1 out]
                n112 = call <vilib>:"NT Read String.vi"("Name"=w219) -> ("String"=w222:string)  [unwired: 9 in, 1 out]
                n113 = Bundle("Numeric"=w221, "String"=w222) -> (→"Progress":cluster{"Numeric":dbl, "String":string})  [unwired: 1 in]
              }
              frame "" {
                n114 = property on="Progress" class="Clust (strict)"("Visible"=FALSE) -> ()  [unwired: 2 in, 2 out]
                n115 = local write "Test Name"(u16 0) -> ()
              }
            }
            n116 = property on="Test Tree" class="Tree (strict)"("Active Item Row Number"=w216, "ActiveColNum"=w216, "CellBG"=w213, "Active Item Row Number"=-1 ("Active Item:Row Number"), "CellBG"=u32 5789784 ("Color Box")) -> ()  [unwired: 2 in, 2 out]
          }
          frame "Variables" {
            w228 = string[] ["CameraPublisher", "Usage", "DB"]  # Items to initially close
            n117 = First Call?() -> (First Call?: T/F=w229:bool)
            n118 = control-ref of="Tree"() -> (w230:refnum<vi>)
            n119 = Select(t=w228, s=w229, f=string[] []) -> (s? t:f=w226:string[])
            n120 = call <vilib>:"NT Read and Format Entries as Tree.vi"("Tags to  Close"=w226, "Tree Refnum"=w230) -> ()  [unwired: 8 in, 2 out]
          }
          frame "Commands" {
            w239 = u32 5789784 ("Color Box")
            w240 = T30 {"Row"=-1, "Column"=-2} ("Active Cell:Active Cell")
            w242 = T30 {"Row"=-2, "Column"=-2} ("Active Cell:Active Cell")
            n121 = Index Array(array=w243, index=w237) -> (element=w241:u32)
            n122 = Index Array(array=w238, index=w237) -> (element=w236:T29)
            n123 = Unbundle(w236) -> ("Operation"=w235:enum16{"Update", "Clear"})  [unwired: 1 out]
            n124 = local read "Command Selection"() -> (w234:i32)
            n125 = property on="Command Selection" class="MCListbox (strict)"("ActiveCell"=w242, "CellBG"=w241, "ActiveCell"=w240, "CellBG"=w239) -> ()  [unwired: 2 in, 2 out]
            n126 = call <vilib>:"WPI_DashboardUpdate RPC Info.vi"("Operation"=w235) -> ("update"=w233:bool, "commands"=w232:string[][])  [unwired: 9 in]
            n127 = property on="Command Selection" class="MCListbox (strict)"("ItemNames"=w232) -> ()  [unwired: 2 in, 2 out]
            n128 = property on="Command Params" class="Tbl (strict)"("Active Cell"=w242, "Cell BG Color"=w241, "Active Cell"=w240, "Cell BG Color"=w239) -> ()  [unwired: 2 in, 2 out]
            n129 = call <vilib>:"WPI_DashboardUpdate Command Params.vi"("Update"=w233, "NewVal"=w234, "Commands"=w232, "Param Tbl"=w231) -> ()  [unwired: 7 in, 1 out]
          }
        }
        n130 = call <vilib>:"Connextion Info.vi"() -> ("Connected"=→"NT Connection":bool)  [unwired: 10 in, 1 out]
      }
      event "Test Tree": Value Change {
        # "Show appropriate\ncontrols"
        n131 = event-data() -> ("CtlRef"=w248:refnum<vi>, "NewVal"=w246:string)  [unwired: 1 in]
        n132 = call <vilib>:"WPI_UtilitiesGetTreeIOName.vi"("NewVal"=w246, "TreeControl in"=w248) -> ("I/O Name"=w249:string)  [unwired: 9 in]
        n133 = case shown="\"Camera\"" w249 {
          selector: w249 -> [_ w256 _ w278 w287 _]
          tunnel: w246 -> [_ _ w275 w277 _ w294]
          tunnel: cluster{string[]}[] [{["640x480", "320x240", "160x120"]}, {["Auto", "Fixed indoor", "Fixed outdoor 1", "Fixed outdoor 2", "Fixed fluorescent 1", "Fixed fluorescent 2", "Hold current"]}, {["Auto", "Flicker-free 50 Hz", "Flicker-free 60 Hz", "Hold current"]}, {["None", "Prioritize frame rate", "Prioritize image quality"]}, {["Monochrome", "Color"]}] -> [_ _ _ _ _ w293]
          frame Default {
            w251 = FALSE ("Visible")
            w250 = FALSE ("Visible")
            n134 = property on="Motor" class="Clust (strict)"("Visible"=w250) -> ()  [unwired: 2 in, 2 out]
            n135 = property on="Test Ring" class="Ring (strict)"("Visible"=w250) -> ()  [unwired: 2 in, 2 out]
            n136 = property on="Rev/Fwd" class="Clust (strict)"("Visible"=w251) -> ()  [unwired: 2 in, 2 out]
            n137 = property on="On/Off" class="Bool (strict)"("Visible"=w251) -> ()  [unwired: 2 in, 2 out]
            n138 = property on="Test Slider" class="Slide (strict)"("Visible"=w251) -> ()  [unwired: 2 in, 2 out]
          }
          frame "Analog Out", "Motor", "PWM" {
            w257 = FALSE ("Visible")
            n139 = case shown="\"Analog Out\"" w256 {
              tunnel: [1.0 ("Value") -1.0 ("Value") 0.0 ("Value")] -> w255
              tunnel: [255.0 ("Value") 1.0 ("Value") 5.0 ("Value")] -> w254
              tunnel: [128.0 ("Value") 0.0 ("Value") 0.0 ("Value")] -> w253
              tunnel: [64.0 ("Value") 0.5 ("Value") 1.0 ("Value")] -> w252
              frame "PWM" {
              }
              frame "Motor", Default {
              }
              frame "Analog Out" {
              }
            }
            n140 = property on="Motor" class="Clust (strict)"("Visible"=TRUE) -> ()  [unwired: 2 in, 2 out]
            n141 = property on="Value" class="Slide (strict)"("Value"=w253, "Scale.Minimum"=w255, "Scale.Maximum"=w254, "Scale.Increment"=w252) -> ()  [unwired: 2 in, 2 out]
            n142 = property on="On/Off" class="Bool (strict)"("Visible"=w257) -> ()  [unwired: 2 in, 2 out]
            n143 = property on="Test Slider" class="Slide (strict)"("Visible"=w257) -> ()  [unwired: 2 in, 2 out]
            n144 = property on="Test Ring" class="Ring (strict)"("Visible"=w257) -> ()  [unwired: 2 in, 2 out]
            n145 = property on="Rev/Fwd" class="Clust (strict)"("Visible"=w257) -> ()  [unwired: 2 in, 2 out]
          }
          frame "Servo" {
            w273 = FALSE ("Visible")
            n146 = call <vilib>:"NT Read Number.vi"("Name"=w275) -> ("Numeric"=w274:dbl)  [unwired: 9 in, 1 out]
            n147 = property on="Test Slider" class="Slide (strict)"("Visible"=TRUE, "Scale.Maximum"=170.0 ("Scale.Range:Maximum")) -> ()  [unwired: 2 in, 2 out]
            n148 = local write "Test Slider"(w274) -> ()
            n149 = property on="Motor" class="Clust (strict)"("Visible"=w273) -> ()  [unwired: 2 in, 2 out]
            n150 = property on="Rev/Fwd" class="Clust (strict)"("Visible"=w273) -> ()  [unwired: 2 in, 2 out]
            n151 = property on="On/Off" class="Bool (strict)"("Visible"=w273) -> ()  [unwired: 2 in, 2 out]
            n152 = property on="Test Ring" class="Ring (strict)"("Visible"=w273) -> ()  [unwired: 2 in, 2 out]
          }
          frame "Relay", "Solenoid" {
            w276 = FALSE ("Visible")
            n153 = property on="Motor" class="Clust (strict)"("Visible"=w276) -> ()  [unwired: 2 in, 2 out]
            n154 = property on="Test Slider" class="Slide (strict)"("Visible"=w276) -> ()  [unwired: 2 in, 2 out]
            n155 = Search and Replace String(input string=w277, search string="/Value  **", replace string="/Direction") -> (result string=w283:string)  [unwired: 5 in, 3 out]
            n156 = property on="Test Ring" class="Ring (strict)"("Visible"=w276) -> ()  [unwired: 2 in, 2 out]
            n157 = call <vilib>:"NT Read String.vi"("Name"=w283) -> ("String"=w281:string)  [unwired: 9 in, 1 out]
            n158 = Equal?(x="Both directions", y=w281) -> (x = y?=w279:bool)
            n159 = Not(x=w279) -> (.not. x?=w280:bool)
            n160 = property on="Rev/Fwd" class="Clust (strict)"("Visible"=w279) -> ()  [unwired: 2 in, 2 out]
            n161 = property on="On/Off" class="Bool (strict)"("Visible"=w280, "Caption.Text"=w278) -> ()  [unwired: 2 in, 2 out]
          }
          frame "Compressor", "Digital Out" {
            w286 = FALSE ("Visible")
            # "Get direction and finish"
            n162 = property on="Motor" class="Clust (strict)"("Visible"=w286) -> ()  [unwired: 2 in, 2 out]
            n163 = property on="Test Slider" class="Slide (strict)"("Visible"=w286) -> ()  [unwired: 2 in, 2 out]
            n164 = property on="Test Ring" class="Ring (strict)"("Visible"=w286) -> ()  [unwired: 2 in, 2 out]
            n165 = property on="On/Off" class="Bool (strict)"("Visible"=TRUE, "Caption.Text"=w287) -> ()  [unwired: 2 in, 2 out]
            n166 = property on="Rev/Fwd" class="Clust (strict)"("Visible"=FALSE) -> ()  [unwired: 2 in, 2 out]
          }
          frame "Camera" {
            n167 = call <vilib>:"Get Last Path Segment.vi"("String in"=w294) -> ("String out"=w295:string)  [unwired: 10 in]
            n168 = property on="On/Off" class="Bool (strict)"("Visible"=FALSE) -> ()  [unwired: 2 in, 2 out]
            n169 = property on="Motor" class="Clust (strict)"("Visible"=FALSE) -> ()  [unwired: 2 in, 2 out]
            n170 = property on="Rev/Fwd" class="Clust (strict)"("Visible"=FALSE) -> ()  [unwired: 2 in, 2 out]
            n171 = case shown="\"White Balance  **\"" w295 {
              tunnel: w294 -> [w301 w310 w319 w328 w337 _ w343]
              tunnel: w293 -> [w299 w307 w316 w325 w334 _ _]
              frame "Size  **" {
                n172 = Index Array(array=w299) -> (element=w298:cluster{string[]})  [unwired: 1 in]
                n173 = call <vilib>:"NT Read String.vi"("Name"=w301) -> ("String"=w300:string)  [unwired: 9 in, 1 out]
                n174 = Unbundle(w298) -> (w296:string[])
                n175 = Match First String(2:w296, 3:w300) -> (0:w297:i32)  [unwired: 1 out]
                n176 = property on="Test Ring" class="Ring (strict)"("Value"=w297, "Strings []"=w296) -> ()  [unwired: 2 in, 2 out]
                n177 = property on="Test Ring" class="Ring (strict)"("Visible"=TRUE) -> ()  [unwired: 2 in, 2 out]
                n178 = property on="Test Slider" class="Slide (strict)"("Visible"=FALSE) -> ()  [unwired: 2 in, 2 out]
              }
              frame "White Balance  **" {
                n179 = Index Array(array=w307, index=1) -> (element=w308:cluster{string[]})
                n180 = call <vilib>:"NT Read String.vi"("Name"=w310) -> ("String"=w309:string)  [unwired: 9 in, 1 out]
                n181 = Unbundle(w308) -> (w305:string[])
                n182 = Match First String(2:w305, 3:w309) -> (0:w304:i32)  [unwired: 1 out]
                n183 = property on="Test Ring" class="Ring (strict)"("Value"=w304, "Strings []"=w305) -> ()  [unwired: 2 in, 2 out]
                n184 = property on="Test Ring" class="Ring (strict)"("Visible"=TRUE) -> ()  [unwired: 2 in, 2 out]
                n185 = property on="Test Slider" class="Slide (strict)"("Visible"=FALSE) -> ()  [unwired: 2 in, 2 out]
              }
              frame "Exposure  **" {
                n186 = Index Array(array=w316, index=2) -> (element=w317:cluster{string[]})
                n187 = call <vilib>:"NT Read String.vi"("Name"=w319) -> ("String"=w318:string)  [unwired: 9 in, 1 out]
                n188 = Unbundle(w317) -> (w313:string[])
                n189 = Match First String(2:w313, 3:w318) -> (0:w314:i32)  [unwired: 1 out]
                n190 = property on="Test Ring" class="Ring (strict)"("Value"=w314, "Strings []"=w313) -> ()  [unwired: 2 in, 2 out]
                n191 = property on="Test Ring" class="Ring (strict)"("Visible"=TRUE) -> ()  [unwired: 2 in, 2 out]
                n192 = property on="Test Slider" class="Slide (strict)"("Visible"=FALSE) -> ()  [unwired: 2 in, 2 out]
              }
              frame "Exposure Priority  **" {
                n193 = Index Array(array=w325, index=3) -> (element=w326:cluster{string[]})
                n194 = call <vilib>:"NT Read String.vi"("Name"=w328) -> ("String"=w327:string)  [unwired: 9 in, 1 out]
                n195 = Unbundle(w326) -> (w322:string[])
                n196 = Match First String(2:w322, 3:w327) -> (0:w323:i32)  [unwired: 1 out]
                n197 = property on="Test Ring" class="Ring (strict)"("Value"=w323, "Strings []"=w322) -> ()  [unwired: 2 in, 2 out]
                n198 = property on="Test Ring" class="Ring (strict)"("Visible"=TRUE) -> ()  [unwired: 2 in, 2 out]
                n199 = property on="Test Slider" class="Slide (strict)"("Visible"=FALSE) -> ()  [unwired: 2 in, 2 out]
              }
              frame "Color Enable  **" {
                n200 = Index Array(array=w334, index=4) -> (element=w335:cluster{string[]})
                n201 = call <vilib>:"NT Read String.vi"("Name"=w337) -> ("String"=w336:string)  [unwired: 9 in, 1 out]
                n202 = Unbundle(w335) -> (w331:string[])
                n203 = Match First String(2:w331, 3:w336) -> (0:w332:i32)  [unwired: 1 out]
                n204 = property on="Test Ring" class="Ring (strict)"("Value"=w332, "Strings []"=w331) -> ()  [unwired: 2 in, 2 out]
                n205 = property on="Test Ring" class="Ring (strict)"("Visible"=TRUE) -> ()  [unwired: 2 in, 2 out]
                n206 = property on="Test Slider" class="Slide (strict)"("Visible"=FALSE) -> ()  [unwired: 2 in, 2 out]
              }
              frame Default {
                n207 = property on="Test Ring" class="Ring (strict)"("Visible"=FALSE) -> ()  [unwired: 2 in, 2 out]
                n208 = property on="Test Slider" class="Slide (strict)"("Visible"=FALSE) -> ()  [unwired: 2 in, 2 out]
              }
              frame "Brightness  **", "Color Level  **", "Compression  **", "FPS  **", "Sharpness  **" {
                n209 = call <vilib>:"NT Read Number.vi"("Name"=w343) -> ("Numeric"=w342:dbl)  [unwired: 9 in, 1 out]
                n210 = local write "Test Slider"(w342) -> ()
                n211 = property on="Test Slider" class="Slide (strict)"("Visible"=TRUE, "Scale.Maximum"=100.0 ("Scale.Range:Maximum")) -> ()  [unwired: 2 in, 2 out]
                n212 = property on="Test Ring" class="Ring (strict)"("Visible"=FALSE) -> ()  [unwired: 2 in, 2 out]
              }
            }
          }
        }
        n213 = property on="Progress" class="Clust (strict)"("Visible"=FALSE) -> ()  [unwired: 2 in, 2 out]
      }
      event "Test Name": Mouse Enter {
        # "Populate the ring with the list of tests"
        n214 = event-data() -> ()  [unwired: 1 in, 1 out]
        n215 = call <vilib>:"NT Read String Array.vi"("Name"="TestMode/TestList") -> ("String Array"=w351:string[])  [unwired: 9 in, 1 out]
        n216 = Build Array (concatenate)("Select the test to run...", w351) -> (w350:string[])
        n217 = property on="Test Name" class="Ring (strict)"("Strings []"=w350) -> ()  [unwired: 2 in, 2 out]
      }
      event "Test Name": Value Change {
        w353 = FALSE ("Visible")
        # "Tell the robot the test name to run"
        n218 = event-data() -> ("NewVal"=w357:u16)  [unwired: 1 in]
        n219 = property on="Test Name" class="Ring (strict)"() -> ("Strings []"=w358:string[])  [unwired: 2 in, 2 out]
        n220 = local write "Progress"(T9 {"Test Progress"=0, "Test Progress Text"=""} ("Progress")) -> ()
        n221 = Index Array(array=w358, index=w357) -> (element=w356:string)
        n222 = call <vilib>:"NT Write String.vi"("String"=w356, "Name"="TestMode/TestName") -> ()  [unwired: 9 in, 1 out]
        n223 = property on="Progress" class="Clust (strict)"("Visible"=TRUE) -> ()  [unwired: 2 in, 2 out]
        n224 = property on="Motor" class="Clust (strict)"("Visible"=w353) -> ()  [unwired: 2 in, 2 out]
        n225 = property on="Test Slider" class="Slide (strict)"("Visible"=w353) -> ()  [unwired: 2 in, 2 out]
        n226 = property on="On/Off" class="Bool (strict)"("Visible"=w353) -> ()  [unwired: 2 in, 2 out]
        n227 = property on="Rev/Fwd" class="Clust (strict)"("Visible"=w353) -> ()  [unwired: 2 in, 2 out]
        n228 = property on="Test Ring" class="Ring (strict)"("Visible"=w353) -> ()  [unwired: 2 in, 2 out]
      }
      event "Select Auto": Mouse Enter {
        # "Populate the combo box with the list of autonomous options"
        n229 = event-data() -> ()  [unwired: 1 in, 1 out]
        n230 = call <vilib>:"NT Read String Array.vi"("Name"="Auto List") -> ("String Array"=w360:string[])  [unwired: 9 in, 1 out]
        n231 = property on="Select Auto" class="CmbBox"("Strings[]"=w360) -> ()  [unwired: 2 in, 2 out]
      }
      event "Select Auto": Value Change {
        # "User modified the Auto Selection. Write to NT variable so robot knows."
        n232 = event-data() -> ("NewVal"=w363:string)  [unwired: 1 in]
        n233 = call <vilib>:"NT Write String.vi"("String"=w363, "Name"="Auto Selector") -> ()  [unwired: 9 in, 1 out]
      }
      event "Command Selection": Value Change {
        # "Get the params and show in table"
        n234 = event-data() -> ("NewVal"=w369:i32)  [unwired: 1 in]
        n235 = property on="Command Selection" class="MCListbox (strict)"() -> ("ItemNames"=w367:string[][])  [unwired: 2 in, 2 out]
        n236 = call <vilib>:"WPI_DashboardUpdate Command Params.vi"("NewVal"=w369, "Commands"=w367, "Param Tbl"=w368) -> ()  [unwired: 8 in, 1 out]
      }
      event "Execute Command": Value Change {
        # "Started one, Unique ID holds\nresponse"
        n237 = event-data() -> ()  [unwired: 1 in, 1 out]
        n238 = property on="Command Selection" class="MCListbox (strict)"() -> ("ItemNames"=w380:string[][])  [unwired: 2 in, 2 out]
        n239 = Index Array(array=w380, index (row)="Command Selection", index (col)=0) -> (element=w378:string)
        n240 = call <vilib>:"Invoke Commands.vi"("Command Params"="Command Params", "Function Name"=w378) -> ("Params"=w374:u8, "Started"=w373:bool)  [unwired: 7 in, 1 out]
        n241 = Array Subset(array="Command Params", length (row)=w374) -> (w375:string[][])  [unwired: 3 in]
        n242 = Select(t="Executing" ("Cmd Status"), s=w373, f="" ("Cmd Status")) -> (s? t:f=→"Cmd Status":string)
      }
      event "Command Selection": Double Click {
        n243 = event-data() -> ("Row"=w388:i32)  [unwired: 1 in]
        n244 = property on="Command Selection" class="MCListbox (strict)"() -> ("ItemNames"=w391:string[][])  [unwired: 2 in, 2 out]
        n245 = local read "Command Params"() -> (w387:string[][])
        n246 = Index Array(array=w391, index (row)=w388, index (col)=0) -> (element=w389:string)
        n247 = call <vilib>:"Invoke Commands.vi"("Command Params"=w387, "Function Name"=w389) -> ("Params"=w386:u8, "Started"=w381:bool)  [unwired: 7 in, 1 out]
        n248 = Array Subset(array=w387, length (row)=w386) -> (w385:string[][])  [unwired: 3 in]
        n249 = Select(t="Executing" ("Cmd Status"), s=w381, f="" ("Cmd Status")) -> (s? t:f=w382:string)
        n250 = local write "Cmd Status"(w382) -> ()
      }
      event "CheckList": Double Click {
        # "Shift clears all"
        # "Update symbols on the listbox"
        n251 = event-data() -> ("PlatMods.Shift"=w393:bool, "Row"=w395:i32)  [unwired: 1 in]
        n252 = case shown="True" w393 {
          tunnel: w395 -> [w399 _]
          tunnel: 1 -> [w398 _]
          frame False {
            n253 = property on="CheckList" class="LstBox (strict)"() -> ("Item Symbols"=w397:i32[])  [unwired: 2 in, 2 out]
            n254 = Replace Array Subset(array=w397, new element=w398, index=w399) -> (w396:i32[])
            n255 = property on="CheckList" class="LstBox (strict)"("Item Symbols"=w396) -> ()  [unwired: 2 in, 2 out]
          }
          frame True {
            w400 = 0 ("Top Row")
            n256 = property on="CheckList" class="LstBox (strict)"() -> ("Number of Rows"=w402:u32)  [unwired: 2 in, 2 out]
            n257 = Initialize Array(0, w402) -> (w401:i32[])
            n258 = property on="CheckList" class="LstBox (strict)"("Top Row"=w400, "Value"=w400, "Item Symbols"=w401) -> ()  [unwired: 2 in, 2 out]
          }
        }
      }
      event "CheckList": Key Down {
        # "Update symbols on the listbox\nLeft and right keys check and uncheck"
        n259 = event-data() -> ("VKey"=w406:T27)  [unwired: 1 in]
        n260 = case shown="\"Left\", \"Right\"" w406 {
          selector: w406 -> [w411 _]
          tunnel: eventvkey."Left" ("VKey") -> [w409 _]
          frame "Left", "Right" {
            n261 = Equal?(x=w409, y=w411) -> (x = y?=w410:bool)
            n262 = Select(t=0, s=w410, f=1) -> (s? t:f=w412:i32)
            n263 = property on="CheckList" class="LstBox (strict)"() -> ("Item Symbols"=w415:i32[])  [unwired: 2 in, 2 out]
            n264 = Replace Array Subset(array=w415, new element=w412, index="CheckList") -> (w414:i32[])
            n265 = property on="CheckList" class="LstBox (strict)"("Item Symbols"=w414) -> ()  [unwired: 2 in, 2 out]
          }
          frame Default {
          }
        }
      }
      event "Motor.Enable": Value Change {
        # "When the test mode otor enable helper is set, update that\ntree row item's value"
        n266 = event-data() -> ("NewVal"=w421:bool)  [unwired: 1 in]
        n267 = Unbundle("Motor") -> ("Value"=w420:dbl)  [unwired: 1 out]
        n268 = Select(t=w420, s=w421, f=0.0) -> (s? t:f=w418:dbl)
        n269 = call <vilib>:"NT Write Number.vi"("Numeric"=w418, "Name"=w417) -> ()  [unwired: 9 in, 1 out]
      }
      event "Test Slider": Value Change {
        # "When the test mode slider helper is set, update that\ntree row item's value"
        n270 = event-data() -> ("NewVal"=w424:dbl)  [unwired: 1 in]
        n271 = call <vilib>:"NT Write Number.vi"("Numeric"=w424, "Name"=w425) -> ()  [unwired: 9 in, 1 out]
      }
      event "On/Off": Value Change {
        # "When the test mode on/off helper value is set, update that\ntree row item's value"
        n272 = event-data() -> ("NewVal"=w429:bool)  [unwired: 1 in]
        n273 = Boolean To (0,1)(Boolean=w429) -> (0, 1=w428:i16)
        n274 = call <vilib>:"NT Write Number.vi"("Numeric"=w428, "Name"=w427) -> ()  [unwired: 9 in, 1 out]
      }
      event "Rev/Fwd": Value Change {
        # "When the test mode helper value for relays is set, update that\ntree row item's value"
        n275 = event-data() -> ("NewVal.Forward"=w437:bool, "NewVal.Reverse"=w436:bool)  [unwired: 1 in]
        n276 = Boolean To (0,1)(Boolean=w437) -> (0, 1=w433:i16)
        n277 = Boolean To (0,1)(Boolean=w436) -> (0, 1=w435:i16)
        n278 = Negate(x=w435) -> (-x=w434:i16)
        n279 = Add(x=w433, y=w434) -> (x+y=w432:i16)
        n280 = call <vilib>:"NT Write Number.vi"("Numeric"=w432, "Name"=w431) -> ()  [unwired: 9 in, 1 out]
      }
      event "Test Ring": Value Change {
        # "When a test mode helper value is selected from the ring,\nset the tree item's variable to the string value"
        n281 = event-data() -> ("NewVal"=w441:u16)  [unwired: 1 in]
        n282 = property on="Test Ring" class="Ring (strict)"() -> ("Strings []"=w442:string[])  [unwired: 2 in, 2 out]
        n283 = Index Array(array=w442, index=w441) -> (element=w440:string)
        n284 = call <vilib>:"NT Write String.vi"("String"=w440, "Name"=w439) -> ()  [unwired: 9 in, 1 out]
      }
      event "Rec Mode": Value Change {
        # "Update globals for recording mode and path to read log from.\nClear when logging and let NetworkTables set path for vision to\nuse."
        n285 = event-data() -> ("NewVal"=w453:enum32{"Stop", "Record", "Playback"})  [unwired: 1 in]
        n286 = global write "WPI_DashboardLogging Global.vi" "Logging Filename"(path "") -> ()
        n287 = global write "WPI_DashboardLogging Global.vi" "Recording"(w453) -> ()
        n288 = case shown="\"Playback\"" w453 {
          tunnel: w452 -> [_ w455 w464]
          tunnel: [_ _ w463] -> w450
          tunnel: [_ _ w462] -> _
          tunnel: w448 -> [_ _ w460]
          tunnel: cluster{i32, i32} {-250, 170} -> [_ _ w459]
          tunnel: [_ _ T28 {"Image Size"=TRUE, "Image Type"=TRUE, "Pixel Value"=TRUE, "ROI Information"=TRUE, "Zoom Factor"=FALSE} ("Image Information Shown:All Elements")] -> w443
          tunnel: [_ _ TRUE ("Zoom Factor")] -> w444
          tunnel: w446 -> [_ _ w456]
          frame Default {
          }
          frame "Stop", "Record" {
            # "Place Window too"
            n289 = invoke class="VI" method="FP.Close"(reference=w455) -> (reference out=w454:refnum<vi>)  [unwired: 2 in, 2 out]
            n290 = invoke class="VI" method="Abort VI"(reference=w454) -> ()  [unwired: 2 in, 3 out]
          }
          frame "Playback" {
            n291 = call "Open Playback Panel.vi"("Offset"=w459, "DB VI Ref"=w460, "Playback in"=w464) -> ("Playback out"=w461:refnum<vi>)  [unwired: 8 in]
            n292 = register-events(w461, w456) -> (reference out=w463:refnum<event-registration>, error out=w462:errorcluster)  [unwired: 2 in]
          }
        }
        n293 = property on="Camera Image Right" class="ImageControl"("Image Information Shown"=w443, "Image Information Visible"=w444) -> ()  [unwired: 2 in, 2 out]
        n294 = property on="Camera Image" class="ImageControl"("Image Information Shown"=w443, "Image Information Visible"=w444) -> ()  [unwired: 2 in, 2 out]
        n295 = call <vilib>:"WPI_DashboardNT Log FieldName Cache.vi"("Operation"=enum16{"Lookup/Add", "Index", "Clear"}."Clear") -> ()  [unwired: 8 in, 3 out]
      }
      event Panel Close {
        w466 = enum32{"Stop", "Record", "Playback"}."Stop" ("Rec Mode")
        # "Playback window has been closed, abort"
        n296 = event-data() -> ()  [unwired: 1 in, 4 out]
        n297 = local write "Rec Mode"(w466) -> ()
        n298 = global write "WPI_DashboardLogging Global.vi" "Recording"(w466) -> ()
      }
      event Panel Close {
        # "Abort playback window and ourself"
        n299 = event-data() -> ()  [unwired: 1 in, 4 out]
        n300 = invoke class="VI" method="FP.Close"(reference=w470) -> (reference out=w469:refnum<vi>)  [unwired: 2 in, 2 out]
        n301 = invoke class="VI" method="Abort VI"(reference=w469) -> (error out=w468:errorcluster)  [unwired: 2 in, 2 out]
        n302 = invoke class="VI" method="Abort VI"(error in=w468) -> ()  [unwired: 2 in, 3 out]
      }
      event User Event {
        n303 = event-data() -> ("IDs"=w477:cluster{"RPC field ID":u16, "Unique ID":u16}, "String"=w476:string)  [unwired: 1 in]
        n304 = Bundle("IDs"=w477, "String"=w476) -> (w475:T14)  [unwired: 1 in]
        n305 = call <vilib>:"Retrieve RPC Response.vi"("RPC Response"=w475) -> ("Output"=w473:string[][])  [unwired: 10 in]
        n306 = Build Array (concatenate)(w471, w473) -> (w472:string[][])
        n307 = local write "Command Params"(w472) -> ()
        n308 = local write "Cmd Status"("" ("Cmd Status")) -> ()
      }
      event "Tree": Double Click {
        n309 = event-data() -> ("PlatMods"=w483:T31, "Tag"=w480:string)  [unwired: 1 in]
        n310 = Unbundle(w483) -> ("Shift"=w482:bool)  [unwired: 4 out]
        n311 = String Subset(string=w480, length (rest)=1 ("length (rest)")) -> (substring=w479:string)  [unwired: 1 in]
        n312 = Not(x=w482) -> (.not. x?=w481:bool)
        n313 = case shown="\"/\"" w479 {
          tunnel: w480 -> [_ w486]
          tunnel: w481 -> [_ w485]
          frame Default {
          }
          frame "/" {
            n314 = call <vilib>:"NT Update Persistence.vi"("Persistence"=w485, "Name"=w486) -> ()  [unwired: 9 in, 1 out]
          }
        }
      }
    }
  }
  n315 = while {
    tunnel: w68 -> [w488]
    i -> [w491]
    stop <- FALSE stop-if-true
    n316 = Wait (ms)(milliseconds to wait=u32 100) -> ()  [unwired: 1 out]
    n317 = case shown="\"Playback\"" "Rec Mode" {
      tunnel: w491 -> [_ _ w506]
      tunnel: [u32 2829099 ("Base Color") u32 11141120 ("Target Color") w495] -> w487
      frame "Stop", Default {
        # "Reset the color, extra updates don't cost much"
      }
      frame "Record" {
      }
      frame "Playback" {
        # "Playback"
        n318 = Quotient & Remainder(x=w506, y=u32 50 ("milliseconds to wait")) -> (x-y*floor(x/y)=w502:u32)  [unwired: 1 out]
        n319 = Divide(x=w502, y=u32 50 ("milliseconds to wait")) -> (x/y=w499:dbl)
        n320 = Multiply(x=6.283185307179586, y=w499) -> (x*y=w504:dbl)
        n321 = Sine(x=w504) -> (sin(x)=w503:dbl)
        n322 = Absolute Value(x=w503) -> (abs(x)=w496:dbl)
        n323 = call "Interpolate RGB Color.vi"("Proportion"=w496, "Target Color"=u32 30976, "Base Color"=u32 2829099) -> ("Result Color"=w495:u32)  [unwired: 8 in]
      }
    }
    n324 = property class="Pane"(reference=w488, "PaneColor"=w487) -> ()  [unwired: 1 in, 2 out]
  }
  n325 = local write "Dashboard Tab"(T13."Camera" ("Dashboard Tab")) -> ()
  n326 = property on="On/Off" class="Bool (strict)"("Visible"=w39) -> ()  [unwired: 2 in, 2 out]
  n327 = property on="Motor" class="Clust (strict)"("Visible"=w39) -> ()  [unwired: 2 in, 2 out]
  n328 = property on="Progress" class="Clust (strict)"("Visible"=w39) -> ()  [unwired: 2 in, 2 out]
  n329 = property on="Test Ring" class="Ring (strict)"("Visible"=w39) -> ()  [unwired: 2 in, 2 out]
  n330 = property on="Rev/Fwd" class="Clust (strict)"("Visible"=w39) -> ()  [unwired: 2 in, 2 out]
  n331 = while {
    tunnel: u16 1741 ("timeout ms (25000)") -> [w508]
    stop <- FALSE stop-if-true
    n332 = TCP Create Listener(10:w508) -> (0:w507:errorcluster, 3:w509:refnum<k5>)  [unwired: 4 in, 1 out]
    n333 = case shown="No Error" w507 {
      selector: w507 -> [w511 _]
      tunnel: w509 -> [w512 _]
      frame No Error {
        n334 = while {
          tunnel: w512 -> [w515]
          tunnel: w511 -> [w514]
          stop <- FALSE stop-if-true
          n335 = TCP Wait On Listener(8:w514, 11:w515) -> (0:w516:errorcluster, 4:w517:refnum<k5>)  [unwired: 2 in, 3 out]
          n336 = local write "TCP"(w517) -> ()
          n337 = case shown="No Error" w516 {
            frame No Error {
            }
            frame Error {
              n338 = Wait (ms)(milliseconds to wait=u32 1000) -> ()  [unwired: 1 out]
            }
          }
        }
      }
      frame Error {
        n339 = Wait (ms)(milliseconds to wait=u32 1000) -> ()  [unwired: 1 out]
      }
    }
  }
  n340 = local write "Command Selection"(u16 0 ("milliseconds to wait")) -> ()
  n341 = local write "Command Params"(string[][] [] ("Command Params")) -> ()
  n342 = global write "WPI_DashboardLogging Global.vi" "Recording"(w62) -> ()
  n343 = local write "Rec Mode"(w62) -> ()
  n344 = call <vilib>:"NT Write String.vi"("String"="Select Auto", "Name"="Auto Selector") -> ()  [unwired: 9 in, 1 out]
